vi "Get Registration.vi"(11 "Event in":refnum<class "Event.lvclass">) -> (2 "Registration":refnum<event-registration>)   [LabVIEW 2021, in "jettl.lvlib" / "Event.lvclass"]
uses:
  Event.lvclass
  Msg Strategy/Msg Strategy.lvclass
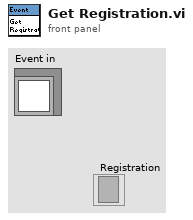
[diagram p1: front panel]
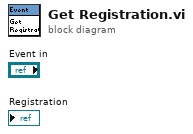
[diagram p0: block diagram]
diagram:
